vi "SUB_FitROI.vi"(5 "Array":u32[](array[numeric]), 7 "Lower":i16, 8 "Upper":i16) -> (0 "Net":i32, 1 "centroid":dbl, 2 "FWHM":dbl, 3 "Integral":i32, 4 "sum":dbl)   [LabVIEW 2015]
uses:
  <vilib>/Analysis/NI_AALPro.lvlib
panel:
  out "x+1":i16
  out "appended array":i32[](array[numeric])
  out "Waveform Graph 2":dbl[](graph)
  out "subarray":u32[](array[numeric])
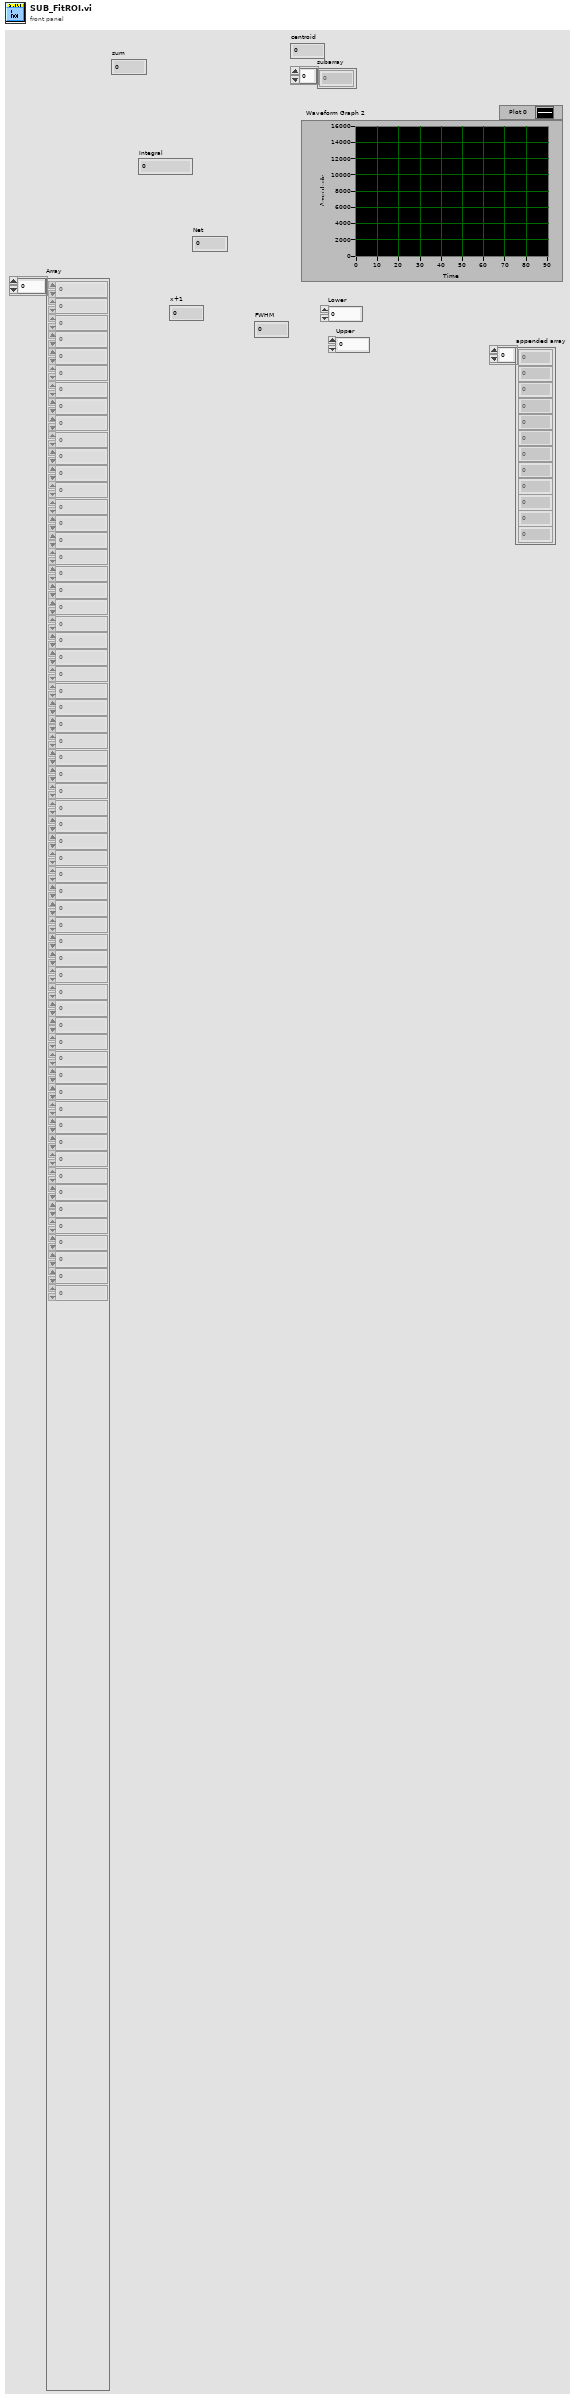
[diagram p1: front panel]
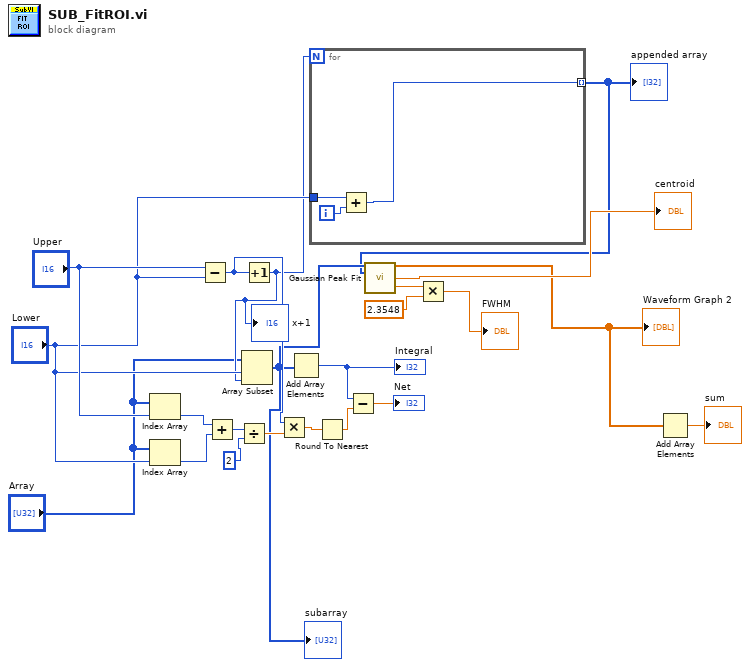
[diagram p0: block diagram]
diagram:
  n1 = Index Array(array="Array", index="Upper") -> (element=w22:u32)
  n2 = Index Array(array="Array", index="Lower") -> (element=w21:u32)
  n3 = Subtract(x="Upper", y="Lower") -> (x-y=w17:i16)
  n4 = Add(x=w22, y=w21) -> (x+y=w20:u32)
  n5 = Divide(x=w20, y=u32 2) -> (x/y=w18:dbl)
  n6 = Increment(x=w17) -> (x+1=w2:i16)
  "x+1" <- w2
  n7 = Array Subset(array="Array", index="Lower", length=w2) -> (w4:u32[])
  "subarray" <- w4
  n8 = Multiply(x=w17, y=w18) -> (x*y=w16:dbl)
  n9 = Add Array Elements(numeric array=w4) -> (sum=w14:u32)
  "Integral" <- w14
  n10 = for {
    N: w2 -> [_]
    tunnel: "Lower" -> [w24]
    tunnel: [w23] -> w3 mode=indexing
    i -> [w25]
    n11 = Add(x=w24, y=w25) -> (x+y=w23:i32)
  }
  "appended array" <- w3
  n12 = Round To Nearest(number=w16) -> (nearest integer value=w15:dbl)
  n13 = Subtract(x=w14, y=w15) -> (x-y=→"Net":dbl)
  n14 = call <vilib>:"Gaussian Peak Fit.vi"("Y"=w4, "X"=w3) -> ("Best Gaussian Fit"=w6:dbl[], "center"=→"centroid":dbl, "standard deviation"=w10:dbl)  [unwired: 7 in, 4 out]
  "Waveform Graph 2" <- w6
  n15 = Multiply(x=w10, y=2.3548) -> (x*y=→"FWHM":dbl)
  n16 = Add Array Elements(numeric array=w6) -> (sum=→"sum":dbl)
